vi "get waveform.vi"(8 "error in (no error)":errorcluster caption="에러 입력(에러 없음)", 11 "Waveform Obj 입력":refnum<class "Waveform Gen.lvclass">) -> (0 "error out":errorcluster caption="에러 출력", 2 "waveform":waveform(dbl), 3 "Waveform Obj 출력":refnum<class "Waveform Gen.lvclass">)   [LabVIEW 2020, in "Waveform Gen.lvclass"]
uses:
  Waveform Gen.lvclass
  Waveform Gen.lvclass/Waveform Gen.ctl
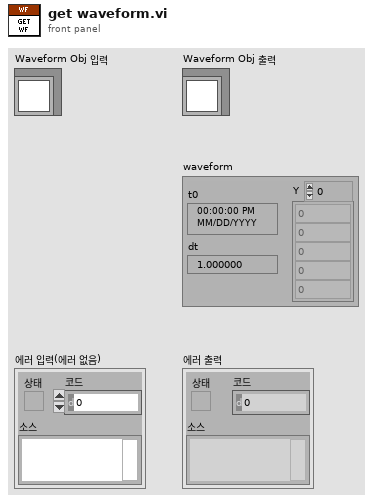
[diagram p1: front panel]
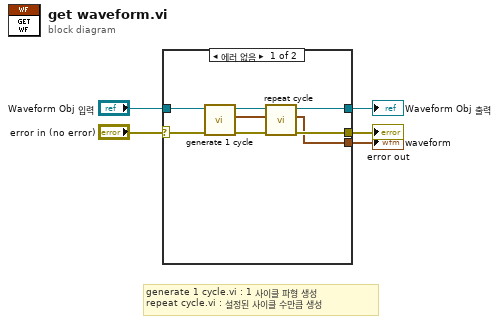
[diagram p0: block diagram]
diagram:
  # "generate 1 cycle.vi : 1 사이클 파형 생성\nrepeat cycle.vi : 설정된 사이클 수만큼 생성"
  n1 = case shown="에러 없음" "error in (no error)" {
    selector: "error in (no error)" -> [w13 w15]
    tunnel: [w7 w15] -> w4
    tunnel: [w8 w14] -> w2
    tunnel: "Waveform Obj 입력" -> [w11 w14]
    tunnel: [w6 _] -> w1
    frame No Error {
      n2 = call-dynamic "generate 1 cycle.vi"("error in (no error)"=w13, "Waveform Obj 입력"=w11) -> ("error out"=w12:errorcluster, "waveform"=w9:waveform(dbl), "Waveform Obj 출력"=w10:refnum<class "Waveform Gen.lvclass">)  [unwired: 7 in]
      n3 = call-dynamic "repeat cycle.vi"("error in (no error)"=w12, "waveform"=w9, "Waveform Obj 입력"=w10) -> ("error out"=w7:errorcluster, "waveform out"=w6:waveform(dbl), "Waveform Obj 출력"=w8:refnum<class "Waveform Gen.lvclass">)  [unwired: 6 in]
    }
    frame Error {
    }
  }
  "error out" <- w4
  "Waveform Obj 출력" <- w2
  "waveform" <- w1
